vi "GUNSC_LibGetAmpsPtr.vi"(8 "error in (no error)":errorcluster) -> (0 "error out":errorcluster, 2 "return value":u64)   [LabVIEW 2014]
uses:
  public/c/lib/libunsc.so
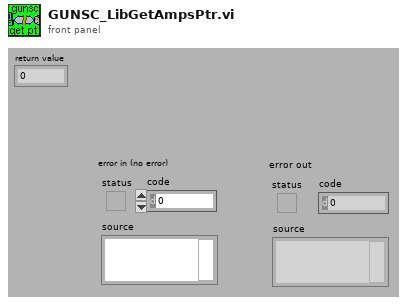
[diagram p1: front panel]
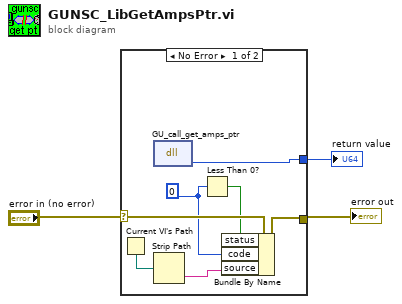
[diagram p0: block diagram]
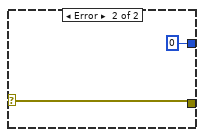
[diagram p2: hidden frame]
diagram:
  n1 = case shown="No Error" "error in (no error)" {
    selector: "error in (no error)" -> [w10 w12]
    tunnel: [w5 0] -> w3
    tunnel: [w6 w12] -> w1
    frame No Error {
      w4 = 0 ("x")
      n2 = Current VI's Path() -> (path=w8:path)
      n3 = dll-call lib="home/sispi/Panview-1.13.0-64b/PAN/Modules/GUNSC/public/c/lib/libunsc.so" fn="GU_call_get_amps_ptr"() -> ("return type"=w5:u64)  [unwired: 3 in, 2 out]
      n4 = Strip Path(path=w8) -> (name=w7:string)  [unwired: 1 out]
      n5 = Less Than 0?(x=w4) -> (x < 0?=w9:bool)
      n6 = Bundle By Name(cluster=w10, "status"=w9, "code"=w4, "source"=w7) -> (w6:errorcluster)
    }
    frame Error {
    }
  }
  "return value" <- w3
  "error out" <- w1
